vi "Main.vi"() -> ()   [LabVIEW 2010]
uses:
  LED Commands.ctl
  Command Classes.ctl
  LvSerial/LvSerial.llb/LvSerial.lvlib
panel:
  in  "Motor Command":bool
  in  "LED 3":bool
  in  "LED 0":bool
  in  "LED 2":bool
  in  "LED 1":bool
  in  "Serial Port":path=path "/dev/ttyUSB0"
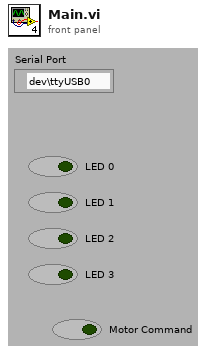
[diagram p1: front panel]
types:
  T1 = typedef "LED Commands.ctl" = enum16{"Enable", "Disable", "Toggle"}
  T2 = typedef "Command Classes.ctl" = enum8{"User Led", "Protocol", "MotorDriver"}
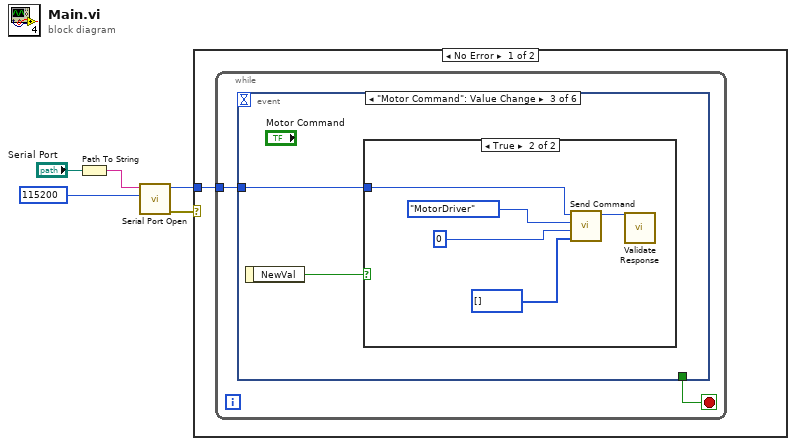
[diagram p0: block diagram]
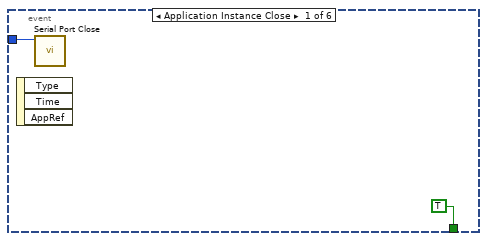
[diagram p2: hidden frame]
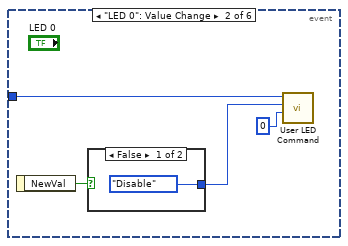
[diagram p3: hidden frame]
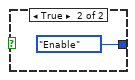
[diagram p4: hidden frame]
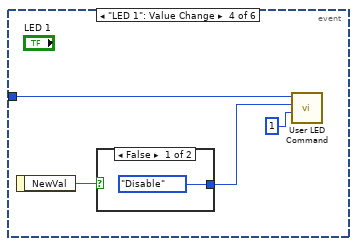
[diagram p6: hidden frame]
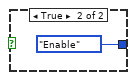
[diagram p7: hidden frame]
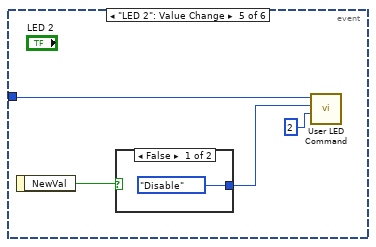
[diagram p8: hidden frame]
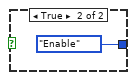
[diagram p9: hidden frame]
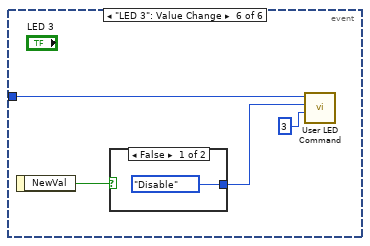
[diagram p10: hidden frame]
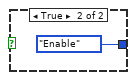
[diagram p11: hidden frame]
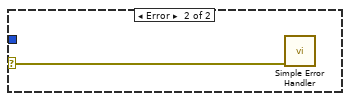
[diagram p12: hidden frame]
diagram:
  n1 = Path To String(path="Serial Port") -> (string=w4:string)
  n2 = call "Serial Port Open.vi"("Baud Rate"=115200, "Port Name"=w4) -> ("Error"=w1:errorcluster, "Port"=w2:i32)  [unwired: 8 in]
  n3 = case shown="No Error" w1 {
    selector: w1 -> [_ w42]
    tunnel: w2 -> [w6 _]
    frame No Error {
      n4 = while {
        tunnel: w6 -> [w8]
        stop <- w7 stop-if-true
        n5 = event shown="[2] \"Motor Command\": Value Change" {
          selector: _ -> [_ _ _ _ _ _]
          dyn-events: _ -> [_ _ _ _ _ _]
          timeout: _ -> [_ _ _ _ _ _]
          tunnel: w8 -> [w10 w14 w17 w25 w31 w37]
          tunnel: [TRUE _ _ _ _ _] -> w7
          event Application Instance Close {
            n6 = event-data() -> ()  [unwired: 1 in, 3 out]
            n7 = call "Serial Port Close.vi"("Port"=w10) -> ()  [unwired: 11 in]
          }
          event "LED 0": Value Change {
            n8 = event-data() -> ("NewVal"=w12:bool)  [unwired: 1 in]
            n9 = case shown="False" w12 {
              tunnel: [LED_Commands."Disable" ("LED Commands") LED_Commands."Enable" ("LED Commands")] -> w11
              frame False {
              }
              frame True {
              }
            }
            n10 = call "User LED Command.vi"("LED Number"=u8 0, "LED Commands"=w11, "Port"=w14) -> ()  [unwired: 7 in, 2 out]
          }
          event "Motor Command": Value Change {
            n11 = event-data() -> ("NewVal"=w18:bool)  [unwired: 1 in]
            n12 = case shown="True" w18 {
              tunnel: w17 -> [_ w23]
              frame False {
              }
              frame True {
                n13 = call "Send Command.vi"("Parameters"=u8[] [], "Command Type"=u8 0, "Command Class"=Command_Classes."MotorDriver", "Port"=w23) -> ("Port"=w19:i32)  [unwired: 7 in]
                n14 = call "Validate Response.vi"("Port"=w19) -> ()  [unwired: 9 in, 2 out]
              }
            }
          }
          event "LED 1": Value Change {
            n15 = event-data() -> ("NewVal"=w24:bool)  [unwired: 1 in]
            n16 = case shown="False" w24 {
              tunnel: [LED_Commands."Disable" ("LED Commands") LED_Commands."Enable" ("LED Commands")] -> w26
              frame False {
              }
              frame True {
              }
            }
            n17 = call "User LED Command.vi"("LED Number"=u8 1, "LED Commands"=w26, "Port"=w25) -> ()  [unwired: 7 in, 2 out]
          }
          event "LED 2": Value Change {
            n18 = event-data() -> ("NewVal"=w30:bool)  [unwired: 1 in]
            n19 = case shown="False" w30 {
              tunnel: [LED_Commands."Disable" ("LED Commands") LED_Commands."Enable" ("LED Commands")] -> w32
              frame False {
              }
              frame True {
              }
            }
            n20 = call "User LED Command.vi"("LED Number"=u8 2, "LED Commands"=w32, "Port"=w31) -> ()  [unwired: 7 in, 2 out]
          }
          event "LED 3": Value Change {
            n21 = event-data() -> ("NewVal"=w36:bool)  [unwired: 1 in]
            n22 = case shown="False" w36 {
              tunnel: [LED_Commands."Disable" ("LED Commands") LED_Commands."Enable" ("LED Commands")] -> w38
              frame False {
              }
              frame True {
              }
            }
            n23 = call "User LED Command.vi"("LED Number"=u8 3, "LED Commands"=w38, "Port"=w37) -> ()  [unwired: 7 in, 2 out]
          }
        }
      }
    }
    frame Error {
      n24 = call <vilib>:"Simple Error Handler.vi"("error in (no error)"=w42) -> ()  [unwired: 4 in, 5 out]
    }
  }
